vi "allAI-temp.vi"(3 "row in":sgl[][](array[numeric]), 4 "array in":sgl[][](array[numeric]), 5 "command":enum16{"get", "set", "clear", "append"}(ring)) -> (0 "range":cluster{"min":sgl, "max":sgl}, 1 "array out":sgl[][](array[numeric]))   [LabVIEW 2015]
panel:
  in  "display":u16(ring)
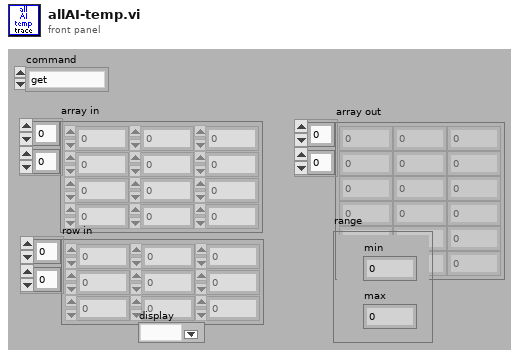
[diagram p1: front panel]
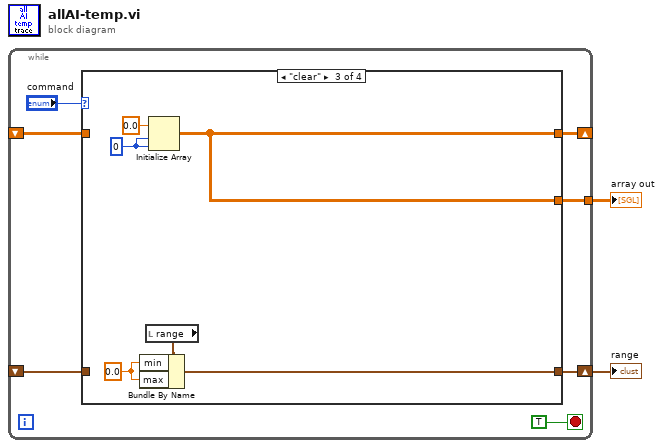
[diagram p0: block diagram]
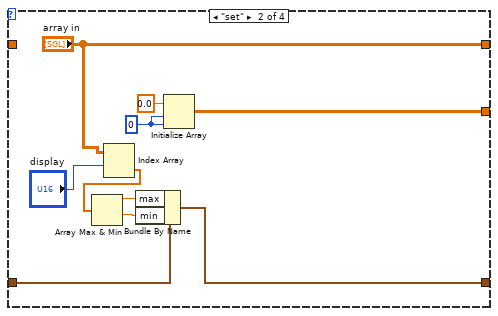
[diagram p3: hidden frame]
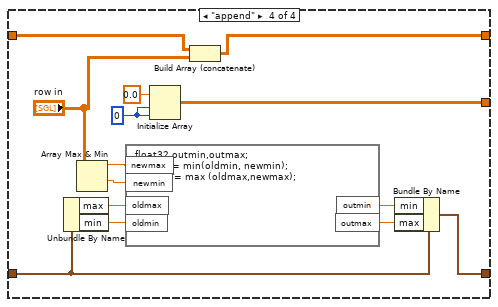
[diagram p4: hidden frame]
diagram:
  n1 = while {
    shift-right: [w7] -> _
    shift-left: _ -> [w8]
    tunnel: [w6] -> w2
    shift-right: [w5] -> w1
    shift-left: _ -> [w4]
    stop <- TRUE stop-if-true
    n2 = case shown="\"clear\"" "command" {
      tunnel: [w11 "array in" w26 w31] -> w7
      tunnel: w8 -> [w11 _ _ w30]
      tunnel: [w11 w20 w26 w40] -> w6
      tunnel: [w10 w16 w23 w32] -> w5
      tunnel: w4 -> [w10 w17 _ w33]
      frame "get", Default {
      }
      frame "set" {
        w15 = 0 ("dimension size")
        n3 = Index Array(array="array in", index (row)="display") -> (element=w12:sgl[])  [unwired: 1 in]
        n4 = Array Max & Min(array=w12) -> (max value=w19:sgl, min value=w18:sgl)  [unwired: 2 out]
        n5 = Bundle By Name(cluster=w17, "max"=w19, "min"=w18) -> (w16:cluster{"min":sgl, "max":sgl})
        n6 = Initialize Array(sgl 0.0 ("element"), w15, w15) -> (w20:sgl[][])
      }
      frame "clear" {
        w24 = sgl 0.0 ("min")
        w22 = 0 ("dimension size")
        n7 = local read "range"() -> (w25:cluster{"min":sgl, "max":sgl})
        n8 = Bundle By Name(cluster=w25, "min"=w24, "max"=w24) -> (w23:cluster{"min":sgl, "max":sgl})
        n9 = Initialize Array(sgl 0.0 ("element"), w22, w22) -> (w26:sgl[][])
      }
      frame "append" {
        w29 = 0 ("dimension size")
        n10 = Unbundle By Name(w33) -> ("max"=w37:sgl, "min"=w36:sgl)
        n11 = Array Max & Min(array="row in") -> (max value=w39:sgl, min value=w38:sgl)  [unwired: 2 out]
        n12 = formula code="float32 outmin,outmax;\noutmin = min(oldmin, newmin);\noutmax = max (oldmax,newmax);"("oldmin"=w36, "oldmax"=w37, "newmax"=w39, "newmin"=w38) -> ("outmin"=w35:sgl, "outmax"=w34:sgl)
        n13 = Initialize Array(sgl 0.0 ("element"), w29, w29) -> (w40:sgl[][])
        n14 = Build Array (concatenate)(w30, "row in") -> (w31:sgl[][])
        n15 = Bundle By Name(cluster=w33, "min"=w35, "max"=w34) -> (w32:cluster{"min":sgl, "max":sgl})
      }
    }
  }
  "array out" <- w2
  "range" <- w1
